vi "Generate Unique Header.vi"(8 "error in":errorcluster, 11 "CRDS Cell Data in":refnum<class "CRDS Cell Data.lvclass">) -> (0 "error out":errorcluster, 2 "Header":string[](array[string]), 3 "CRDS Cell Data out":refnum<class "CRDS Cell Data.lvclass">)   [LabVIEW 2016, in "CRDS Lib.lvlib" / "CRDS Cell Data.lvclass"]
uses:
  CRDS Cell Data.lvclass
  G:/sw_repo/For Builds/Reusable/Data/Data.lvclass
  Data/Data.lvclass/Data.ctl
  CRDS Cell Data.lvclass/CRDS Cell Data.ctl
  Data/Read Data ID.vi
  Read Allan Variances.vi
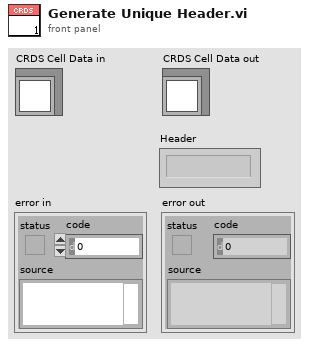
[diagram p1: front panel]
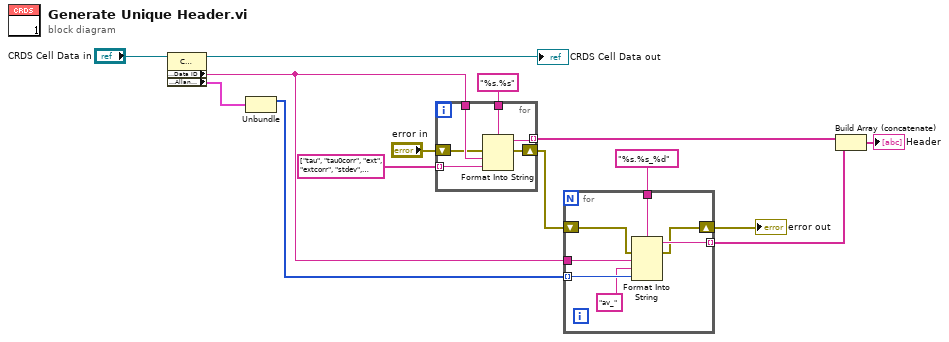
[diagram p0: block diagram]
diagram:
  n1 = property class="CRDS Cell"(reference="CRDS Cell Data in") -> (reference out=→"CRDS Cell Data out":refnum<class "CRDS Cell Data.lvclass">, "Accessors:Data ID"=w7:string, "Data Access:Allan Variances"=w10:cluster{"iTime":i32[], sgl[]})  [unwired: 1 in, 1 out]
  n2 = Unbundle(w10) -> ("iTime"=w9:i32[])  [unwired: 1 out]
  n3 = for {
    tunnel: string[] ["tau", "tau0corr", "ext", "extcorr", "stdev", "etau", "taucorr", "tau0", "max", "rhdilfac", "Q", "Tmean", "extdilfac", "RH", "P", "T"] -> [w20] mode=indexing
    tunnel: [w19] -> w6 mode=indexing
    tunnel: w7 -> [w18]
    tunnel: "%s.%s" ("format string") -> [w17]
    shift-right: [w15] -> w2
    shift-left: "error in" -> [w16]
    n4 = Format Into String(format string=w17, error in=w16, w18, w20) -> (resulting string=w19:string, error out=w15:errorcluster)  [unwired: 1 in]
  }
  n5 = for {
    tunnel: w9 -> [w25] mode=indexing
    tunnel: "%s.%s_%d" ("format string") -> [w27]
    tunnel: w7 -> [w26]
    tunnel: [w23] -> w5 mode=indexing
    shift-right: [w21] -> w1
    shift-left: w2 -> [w22]
    n6 = Format Into String(format string=w27, error in=w22, w26, "av_" ("input 2"), w25) -> (resulting string=w23:string, error out=w21:errorcluster)  [unwired: 1 in]
  }
  "error out" <- w1
  n7 = Build Array (concatenate)(w6, w5) -> (→"Header":string[])
